vi "Add Frames.vi"(7 "Add Info?":bool, 8 "error in (no error)":errorcluster, 9 "Frames":T3[](array[typedef]), 10 "Action":T2, 11 "Section Ref in":T1 format="%.0x") -> (0 "error out":errorcluster, 3 "Section Ref out":T1 format="%.0x")   [LabVIEW 2023, in "J1939 System Definition API Support.lvlib"]
uses:
  J1939 System Definition API Support.lvlib
  Types/Add Item - Frame Cluster.ctl
  Types/Remove Frame Action.ctl
  <vilib>/NI VeriStand/Custom Device API/Custom Device Item Ref.ctl
  Addon/Addon Shared/SubVIs/Constants.vi
  <vilib>/NI/NI VeriStand Advanced SysDef API/_SubVIs/SysDef.Search.GUID.vi
  Addon/Addon Shared/J1939 Addon Shared.lvlib
  <vilib>/NI/NI VeriStand Advanced SysDef API/SysDef API/Advanced System Definition.lvlib
  <vilib>/NI VeriStand/Custom Device API/Custom Device API.lvlib
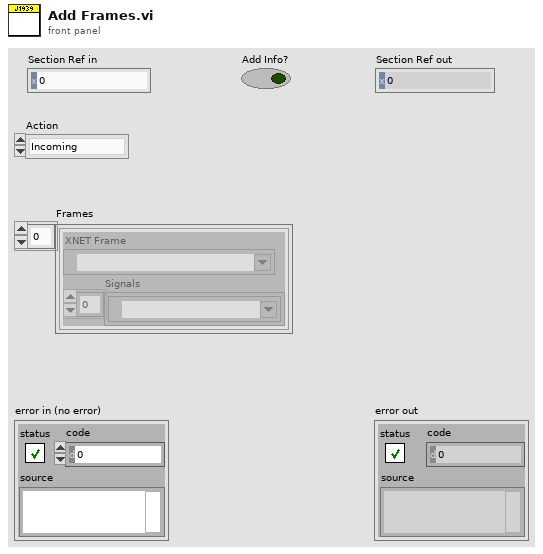
[diagram p1: front panel]
types:
  T1 = typedef "Custom Device API.lvlib/Custom Device Item Ref.ctl" = u64
  T2 = typedef "J1939 System Definition API Support.lvlib/Remove Frame Action.ctl" = enum16{"Incoming", "Outgoing Event", "Outgoing Cyclic", "Outgoing Cyclic Event"}
  T3 = typedef "J1939 System Definition API Support.lvlib/Add Item - Frame Cluster.ctl" = cluster{"XNET Frame":refnum<k21>, "Signals":refnum<k21>[]}
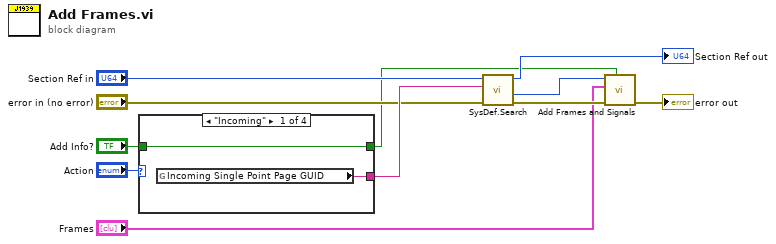
[diagram p0: block diagram]
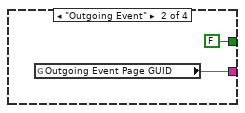
[diagram p2: hidden frame]
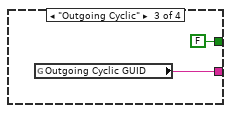
[diagram p3: hidden frame]
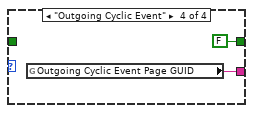
[diagram p4: hidden frame]
diagram:
  n1 = case shown="\"Incoming\"" "Action" {
    tunnel: [w13 w15 w17 w19] -> w6
    tunnel: [w12 FALSE ("Add Info?") FALSE ("Add Info?") FALSE ("Add Info?")] -> w2
    tunnel: "Add Info?" -> [w12 _ _ _]
    frame "Incoming" {
      n2 = global read "Constants.vi" "Incoming Single Point Page GUID"() -> (w13:string)
    }
    frame "Outgoing Event" {
      n3 = global read "Constants.vi" "Outgoing Event Page GUID"() -> (w15:string)
    }
    frame "Outgoing Cyclic" {
      n4 = global read "Constants.vi" "Outgoing Cyclic GUID"() -> (w17:string)
    }
    frame "Outgoing Cyclic Event" {
      n5 = global read "Constants.vi" "Outgoing Cyclic Event Page GUID"() -> (w19:string)
    }
  }
  n6 = call-poly <vilib>:"SysDef.Search.vi"("error in (no error)"="error in (no error)", "GUID"=w6, "nodeID"="Section Ref in") -> ("error out"=w11:errorcluster, "Value out"=w10:u64, "nodeID out"=→"Section Ref out":u64)  [unwired: 5 in, 1 out]
  n7 = call "Add Frames and Signals.vi"("Add Info?"=w2, "error in"=w11, "Frames"="Frames", "Parent Ref in"=w10) -> ("error out"=→"error out":errorcluster)  [unwired: 6 in, 1 out]
